vi "Dashboard Main.vi"() -> ()   [LabVIEW 2012]
uses:
  <vilib>/Rock Robotics/WPI/Camera/WPI_CameraWhite Balance Values.ctl
  <vilib>/event_ctls.llb/eventvkey.ctl
  <vilib>/Utility/config.llb/Read Key (String).vi
  <vilib>/Utility/config.llb/Read Key (I32).vi
  <vilib>/Utility/config.llb/Write Key (String).vi
  <vilib>/Utility/config.llb/Write Key (I32).vi
  <vilib>/Utility/config.llb/NI_LVConfig.lvlib
  <vilib>/Utility/inputDevices.llb/joystickAcquire.vi
panel:
  out "Selected Cordinates":i32[](array[numeric])
  out "Latched Cordinates":i32[](array[numeric])
  out "Battery Value":dbl(slide) scale=0.0..14.0 scale format="%#_2e"
  out "Battery":sgl(graph)
  in  "Camera Settings":T1={"Frate Rate"=30, "Compression"=30, "Size"=1} {"Frate Rate" scale=1.0..30.0; "Size" items=["640x480", "320x240", "160x120"]}
  out "Mode":T2(ring)=enum."Auto Disabled"
  out "Camera IP":string
  out "JS1 Z":dbl(slide) scale=-1.0..1.0 scale format="%#_2e"
  out "JS2 Z":dbl(slide) scale=-1.0..1.0 scale format="%#_2e"
  out "Joystick 1":cluster{"X":dbl, "Y":dbl}[](graph)
  out "Joystick 2":cluster{"X":dbl, "Y":dbl}[](graph)
  out "JS Buttons 1":T3
  out "JS Buttons 2":T3
  out "MotorSlide4":dbl(slide) scale=-1.0..1.0 scale format="%#_2e"
  out "MotorSlide3":dbl(slide) scale=-1.0..1.0 scale format="%#_2e"
  out "MotorSlide2":dbl(slide) scale=-1.0..1.0 scale format="%#_2e"
  in  "MotorName3":string="Front Left"
  in  "MotorName4":string="Front Right"
  in  "MotorName1":string="Rear Left"
  in  "MotorName2":string="Rear Right"
  out "MotorChart4":dbl(graph)
  out "MotorChart3":dbl(graph)
  out "MotorChart2":dbl(graph)
  out "MotorSlide1":dbl(slide) scale=-1.0..1.0 scale format="%#_2e"
  out "MotorChart1":dbl(graph)
  out "Robot IP":string
  in  "Dashboard Tab":enum32{"Operation", "Test", "Checklist"}(tab)
  in  "Checkbox 2":bool
  in  "Checkbox 1":bool
  in  "Slider 1":dbl(slide) scale=0.0..100.0
  in  "Slider":dbl(slide) scale=0.0..100.0 scale format="%#_3g"
  in  "On/Off":bool caption="Solenoid"
  in  "Test Name":u16(ring) items=["Select the test to run...", "Example Test", "-------------------------------", "List of tests is built in robot code.", "Replace with your own automated tests."]
  in  "Test Tree":string(tree)
  in  "Motor":cluster{"Value":dbl, "Enable":bool} {"Value" scale=-1.0..1.0 scale format="%#_3g"}
  out "Progress":T4 {"Test Progress" scale=0.0..100.0}
  in  "Rev/Fwd":cluster{"Forward":bool, "Reverse":bool}
  in  "Ring":u16(ring) items=["Auto", "Fixed indoor", "Fixed outdoor 1", "Fixed outdoor 2", "Fixed fluorescent 1", "Fixed fluorescent 2", "Hold current"]
  in  "Listbox":i32(listbox)
  in  "Viewer":enum32{"Camera Image", "Map", "Variables"}(tab)
  out "Mbps":dbl format="%#.1g"
  in  "Enable":bool
  in  "DB Camera Config":bool
  out "Mbps":bool
  out "fps":dbl format="%#.1g"
  out "Image Error Message":string="Timeout in Camera Communications"
  out "Camera Image":T5(plugin-control)
  out "Map":T5(plugin-control)
  out "Distance [Meter]":dbl
  out "Angel [Degrees]":dbl
  in  "Goal Number":i32(knob) scale=1.0..5.0
  out "Tree":string(tree)
  # "Drive & Motors"
  # "Robot IP:"
  # "Customize by placing controls and indicators here and name to match\nDashboard Variables on robot."
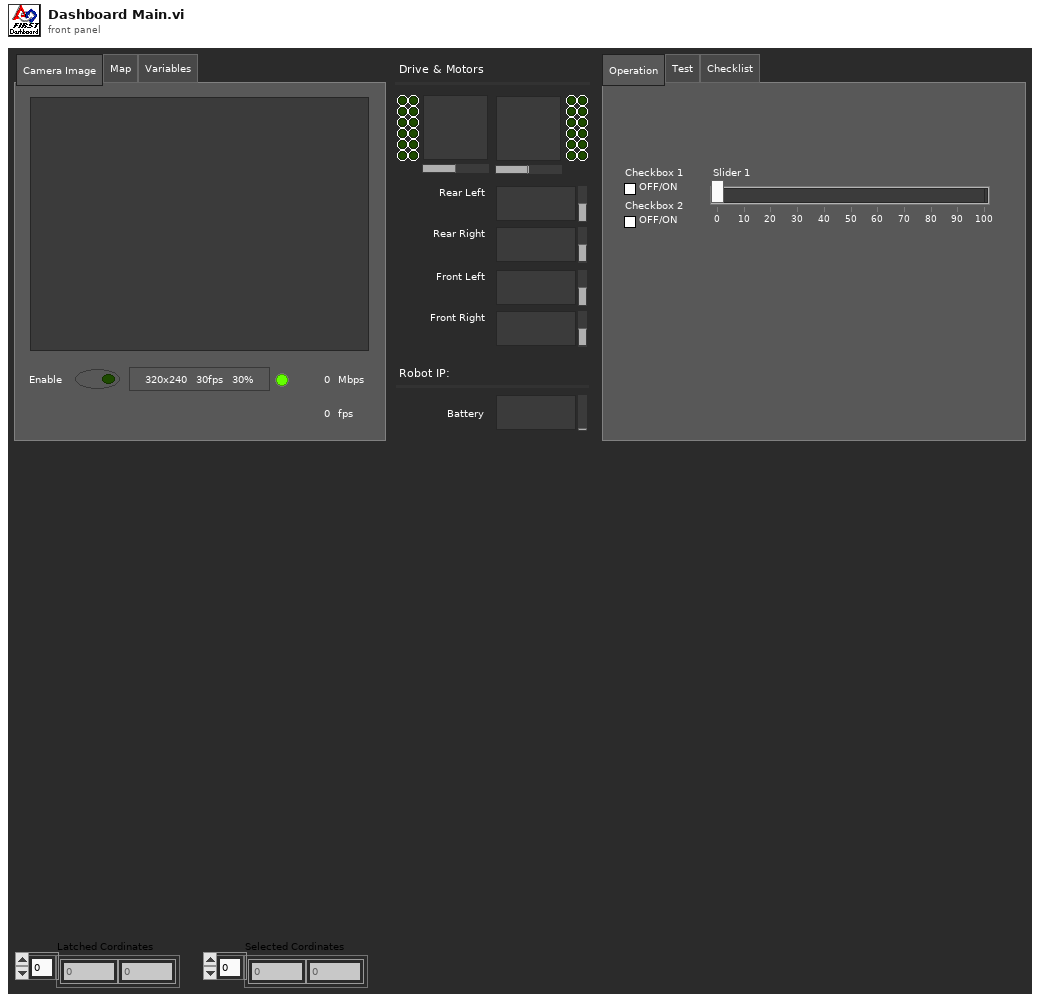
[diagram p1: front panel]
types:
  T1 = cluster{"Frate Rate":i32, "Compression":i32, "Size":u16}
  T2 = enum8{"Tele-Op Disabled", "Tele-Op Enabled", "Auto Disabled", "Auto Enabled", "Test Disabled", "Test Enabled", ""}
  T3 = cluster{bool, bool, bool, bool, bool, bool, bool, bool, bool, bool, bool, bool}
  T4 = cluster{"Test Progress":u8, "Test Progress Text":string}
  T5 = typedef "IMAQ Image.ctl" = refnum<image>
  T6 = typedef "Image Type" = u32
  T7 = typedef "WPI_CameraWhite Balance Values.ctl" = enum16{"Auto", "Fixed indoor", "Fixed outdoor 1", "Fixed outdoor 2", "Fixed fluorescent 1", "Fixed fluorescent 2", "Hold current"}
  T8 = typedef "SkeletonTrackState.ctl" = enum32{"NotTracked", "PositionOnly", "Tracked"}
  T9 = cluster{"TrackingState":u8[], "Position":cluster{"x":sgl, "y":sgl, "z":sgl}, cluster{"x":sgl, "y":sgl, "z":sgl, sgl}[], "TrackState":T8}
  T10 = cluster{cluster{"ScaledToPercentRange":dbl, "ScaledToPercentRange":dbl, "ScaledToPercentRange":dbl}, cluster{bool, bool, bool}}[]
  T11 = cluster{cluster{"ScaledToPercentRange":dbl, "ScaledToPercentRange":dbl, "ScaledToPercentRange":dbl}, cluster{bool, bool, bool}}
  T12 = cluster{"ScaledToPercentRange":dbl, "ScaledToPercentRange":dbl, "ScaledToPercentRange":dbl}
  T13 = typedef "LVRectTypeDef.ctl" = cluster{"Left":i16, "Top":i16, "Right":i16, "Bottom":i16}
  T14 = cluster{"Competition mode":bool, "Robot Link":bool, "Autonomous":bool, "Enabled":bool, "E-Stop":bool, "Simulated":bool, "TestMode":bool, "Docked Window":bool}
  T15 = cluster{"Boolean Array[0]":bool, "Boolean Array[1]":bool, "Boolean Array[2]":bool, "Boolean Array[3]":bool, "Boolean Array[4]":bool, "Boolean Array[5]":bool, "Boolean Array[6]":bool, "Boolean Array[7]":bool, "Boolean Array[8]":bool, "Boolean Array[9]":bool, "Boolean Array[10]":bool, "Boolean Array[11]":bool}
  T16 = cluster{"Coordinates[0]":i32, "Coordinates[1]":i32, "Coordinates[2]":i32, "Coordinates[3]":i32, "Coordinates[4]":i32, "Coordinates[5]":i32, "Coordinates[6]":i32, "Coordinates[7]":i32, "Coordinates[8]":i32}
  T17 = typedef "WPI_CameraDevRef.ctl" = cluster{"Camera Address":string, "CameraStatus":errorcluster, "Acquire Image Notifier":refnum<notifier>}
  T18 = typedef "NI_LVConfig.lvlib/Config Data RefNum.ctl" = refnum<k1>
  T19 = typedef "eventvkey.ctl" = enum16{"ASCII", "Enter", "Return", "Shift", "Ctrl", "Alt", "Cmd", "Opt", "Caps", "NumLock", "Clear", "Break", "Up", "Down", "Left", "Right", "Insert", "Delete", "Home", "End", "PageUp", "PageDown", "Escape", "Help", "Pause", "ScrollLock", "F1", "F2", "F3", "F4", "F5", "F6", "F7", "F8", "F9", "F10", "F11", "F12", "F13", "F14", "F15", "F16", "F17", "F18", "F19", "F20", "F21", "F22", "F23", "F24", "Play", "VolumeUp", "VolumeDown", "Mute", "Two Byte Char"}
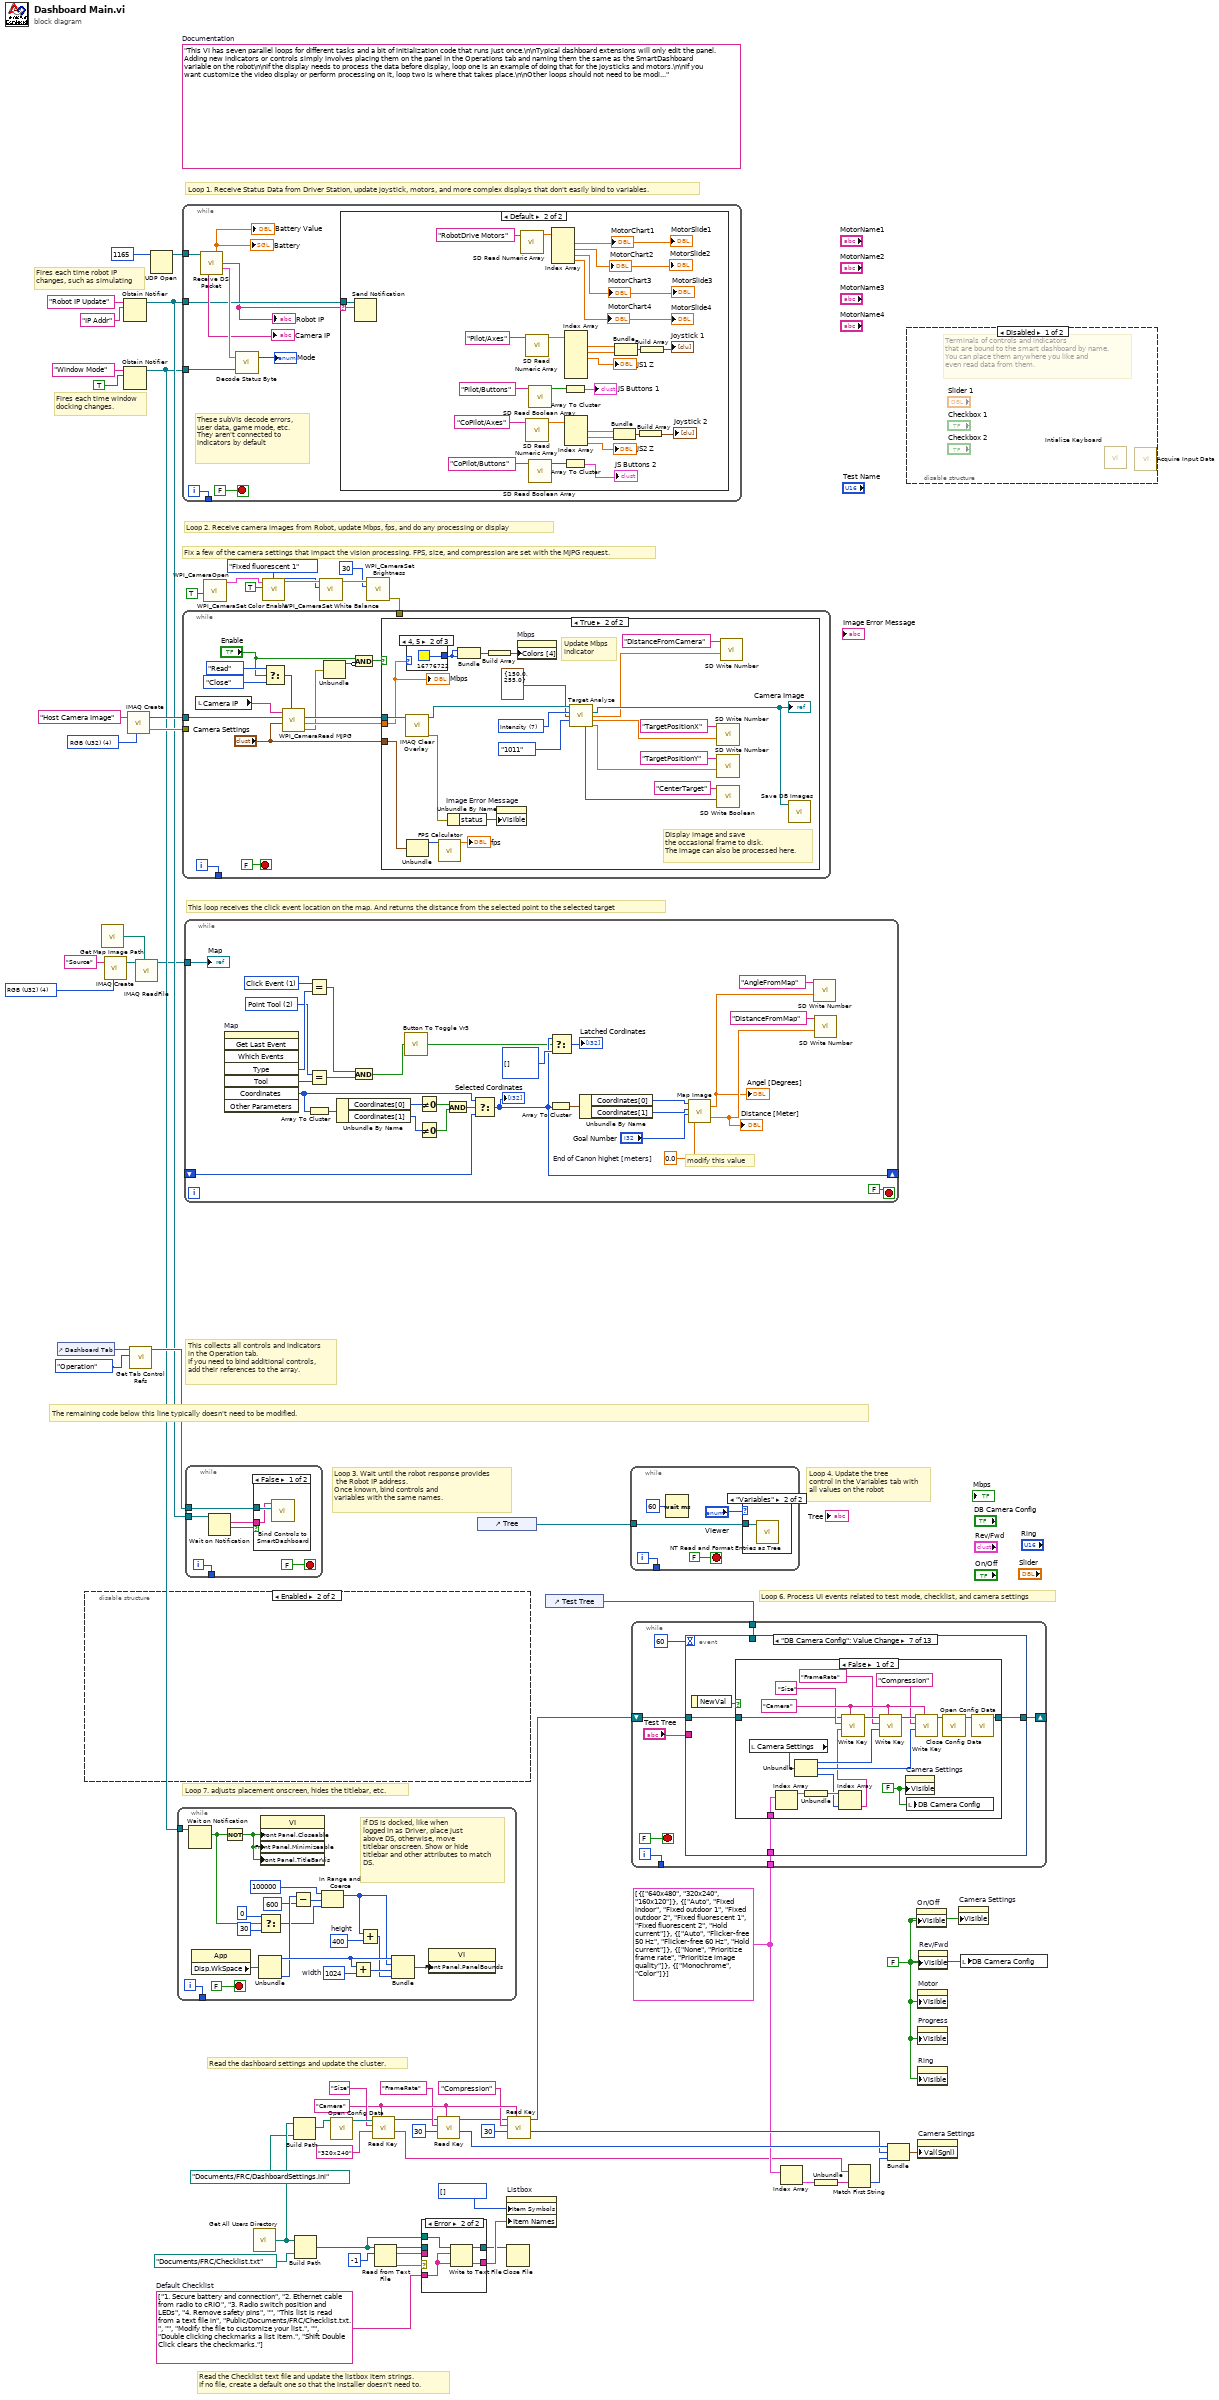
[diagram p0: block diagram]
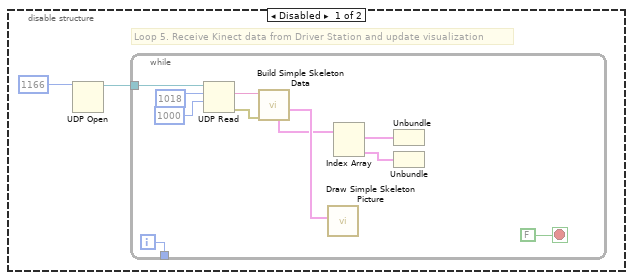
[diagram p2: hidden frame]
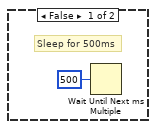
[diagram p5: hidden frame]
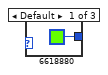
[diagram p6: hidden frame]
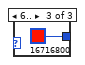
[diagram p7: hidden frame]
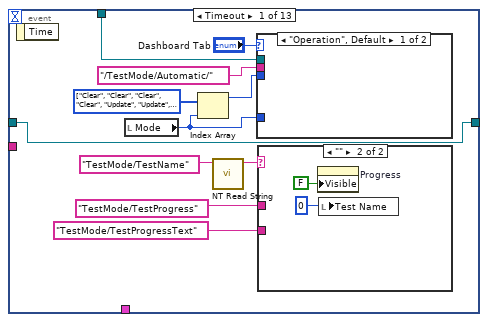
[diagram p9: hidden frame]
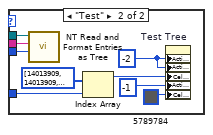
[diagram p10: hidden frame]
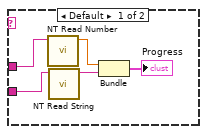
[diagram p11: hidden frame]
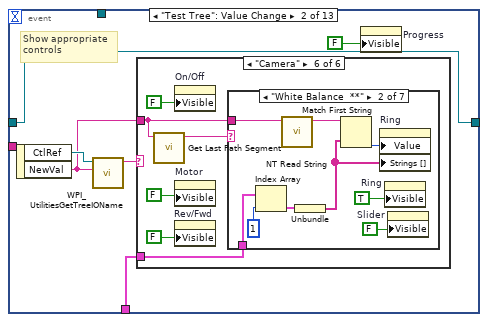
[diagram p12: hidden frame]
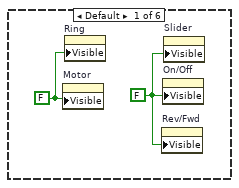
[diagram p13: hidden frame]
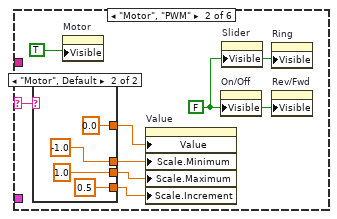
[diagram p14: hidden frame]
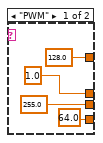
[diagram p15: hidden frame]
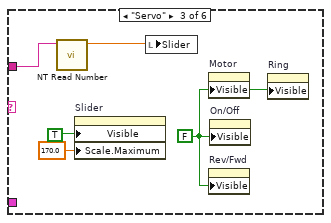
[diagram p16: hidden frame]
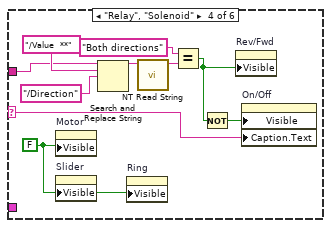
[diagram p17: hidden frame]
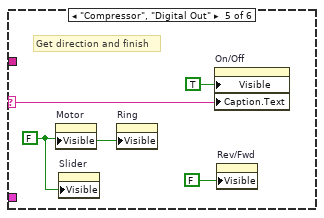
[diagram p18: hidden frame]
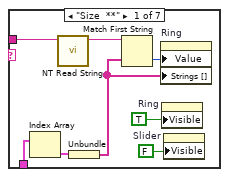
[diagram p19: hidden frame]
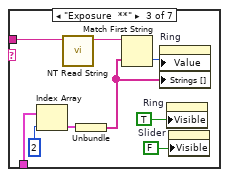
[diagram p20: hidden frame]
diagram:
  w5 = T6 4 items=["Grayscale (U8)", "Grayscale (I16)", "Grayscale (SGL)", "Complex (CSG)", "RGB (U32)", "HSL (U32)", "RGB (U64)", "Grayscale (U16)"] ("Image Type")
  w34 = "Camera"
  w26 = cluster{string[]}[] [{["640x480", "320x240", "160x120"]}, {["Auto", "Fixed indoor", "Fixed outdoor 1", "Fixed outdoor 2", "Fixed fluorescent 1", "Fixed fluorescent 2", "Hold current"]}, {["Auto", "Flicker-free 50 Hz", "Flicker-free 60 Hz", "Hold current"]}, {["None", "Prioritize frame rate", "Prioritize image quality"]}, {["Monochrome", "Color"]}]
  w42 = string[] ["1. Secure battery and connection", "2. Ethernet cable from radio to cRIO", "3. Radio switch position and LEDs", "4. Remove safety pins", "", "This list is read from a text file in", "Public/Documents/FRC/Checklist.txt.", "", "Modify the file to customize your list.", "", "Double clicking checkmarks a list item.", "Shift Double Click clears the checkmarks."]  # Default Checklist
  w40 = FALSE ("Visible")
  (unwired) "This VI has seven parallel loops for different tasks and a bit of initialization code that runs just once.\n\nTypical dashboard extensions will only edit the panel. Adding new indicators or controls simply involves placing them on the panel in the Operations tab and naming them the same as the SmartDashboard variable on the robot\n\nIf the display needs to process the data before display, loop one is an example of doing that for the joysticks and motors.\n\nIf you want customize the video display or perform processing on it, loop two is where that takes place.\n\nOther loops should not need to be modified. They are pretty standard, and document the task they perform."  # Documentation
  w61 = T6 4 items=["Grayscale (U8)", "Grayscale (I16)", "Grayscale (SGL)", "Complex (CSG)", "RGB (U32)", "HSL (U32)", "RGB (U64)"] ("Image Type")
  # "This loop receives the click event location on the map. And returns the distance from the selected point to the selected target"
  # "Fix a few of the camera settings that impact the vision processing. FPS, size, and compression are set with the MJPG request."
  # "Fires each time robot IP\nchanges, such as simulating"
  # "Fires each time window\ndocking changes."
  # "Read the Checklist text file and update the listbox item strings.\nIf no file, create a default one so that the installer doesn't need to."
  # "This collects all controls and indicators\nin the Operation tab.\nIf you need to bind additional controls,\nadd their references to the array."
  # "The remaining code below this line typically doesn't need to be modified."
  # "Loop 6. Process UI events related to test mode, checklist, and camera settings"
  # "Read the dashboard settings and update the cluster."
  # "Loop 4. Update the tree\ncontrol in the Variables tab with\nall values on the robot"
  # "Loop 3. Wait until the robot response provides\n the Robot IP address.\nOnce known, bind controls and\nvariables with the same names."
  # "Loop 7. adjusts placement onscreen, hides the titlebar, etc."
  # "Loop 1. Receive Status Data from Driver Station, update joystick, motors, and more complex displays that don't easily bind to variables."
  # "Loop 2. Receive camera images from Robot, update Mbps, fps, and do any processing or display"
  n1 = control-ref of="Dashboard Tab"() -> (w56:refnum<vi>)
  n2 = disable-structure shown="Enabled" {
    frame Disabled {
      # "Loop 5. Receive Kinect data from Driver Station and update visualization"
      n3 = UDP Open(11:u16 1166 ("port")) -> (port=w64:refnum<k16>)  [unwired: 2 in, 4 out]
      n4 = while {
        tunnel: w64 -> [w80]
        tunnel: [w67] -> _
        i -> [w67]
        stop <- FALSE stop-if-true
        n5 = UDP Read(connection ID=w80, max size (548)=1018 ("bytes to read"), timeout ms (25000)=1000) -> (data out=w75:string, error out=w66:errorcluster)  [unwired: 1 in, 3 out]
        n6 = call "Build Simple Skeleton Data.vi"("error in (no error)"=w66, "data in"=w75) -> ("Skeleton Data"=w76:T9, "NumPlayers"=w78:i8, "Version String"=w79:string, "Simple Joystick Info"=w73:T10)  [unwired: 5 in, 1 out]
        n7 = call "Draw Simple Skeleton Picture.vi"("Simple Skeleton"=w76) -> ("new picture out"=w77:picture)  [unwired: 10 in]
        n8 = Index Array(array=w73) -> (element #1=w72:T11, element #2=w71:T11)  [unwired: 2 in]
        n9 = Unbundle(w72) -> (w70:T12)  [unwired: 1 out]
        n10 = Unbundle(w71) -> (w69:T12, w68:cluster{bool, bool, bool})
      }
    }
    frame Enabled {
    }
  }
  n11 = call "Get Map Image Path.vi"() -> ("Image Path"=w1:path)  [unwired: 1 in]
  n12 = call "IMAQ Create"("Image Name"="Source", "Image Type"=w5) -> ("New Image"=w3:T5)  [unwired: 2 in, 2 out]
  n13 = Obtain Notifier(name (unnamed)="Robot IP Update", notification data type="IP Addr" ("name (unnamed)")) -> (notifier out=w53:refnum<notifier>)  [unwired: 2 in, 2 out]
  n14 = Obtain Notifier(name (unnamed)="Window Mode", notification data type=TRUE) -> (notifier out=w46:refnum<notifier>)  [unwired: 2 in, 2 out]
  n15 = call "IMAQ Create"("Image Name"="Host Camera Image", "Image Type"=w61) -> ("New Image"=w59:T5, "error out"=w58:errorcluster)  [unwired: 2 in, 1 out]
  n16 = call <vilib>:"Get Tab Control Refs.vi"("Page Index"=enum32{"Operation", "Test"}."Operation" ("Dashboard Tab"), "TabControl in"=w56) -> ("ControlsOnPage"=w57:refnum<vi>[])  [unwired: 9 in]
  n17 = call "IMAQ ReadFile"("File Path"=w1, "Image"=w3) -> ("Image Out"=w4:T5)  [unwired: 5 in, 4 out]
  n18 = UDP Open(11:u16 1165 ("port")) -> (port=w62:refnum<k16>)  [unwired: 2 in, 4 out]
  n19 = while {
    tunnel: w46 -> [w101]
    tunnel: [w99] -> _
    i -> [w99]
    stop <- FALSE stop-if-true
    w91 = 1024  # width
    w94 = 400  # height
    # "If DS is docked, like when\nlogged in as Driver, place just\nabove DS, otherwise, move\ntitlebar onscreen. Show or hide\ntitlebar and other attributes to match\nDS."
    n20 = Wait on Notification(notifier=w101) -> (notification=w86:bool)  [unwired: 3 in, 3 out]
    n21 = property class="App"() -> ("Disp.WkSpace"=w97:T13)  [unwired: 2 in, 2 out]
    n22 = Not(x=w86) -> (.not. x?=w100:bool)
    n23 = Unbundle(w97) -> ("Left"=w95:i16, "Bottom"=w92:i16)  [unwired: 2 out]
    n24 = Select(t=0, s=w86, f=30) -> (s? t:f=w85:i32)
    n25 = property class="VI"("Front Panel.Closeable"=w100, "Front Panel.Minimizeable"=w100, "Front Panel.TitleBarVis"=w100) -> ()  [unwired: 2 in, 2 out]
    n26 = Subtract(x=w92, y=600) -> (x-y=w89:i32)
    n27 = In Range and Coerce(upper limit=100000, x=w89, lower limit=w85) -> (coerced(x)=w83:i32)  [unwired: 1 out]
    n28 = Add(x=w95, y=w91) -> (x+y=w96:i32)
    n29 = Add(x=w83, y=w94) -> (x+y=w93:i32)
    n30 = Bundle("Left"=w95, w83, w96, w93) -> (w98:cluster{"Left":i16, i32, i32, i32})  [unwired: 1 out]
    n31 = property class="VI"("Front Panel.PanelBounds"=w98) -> ()  [unwired: 2 in, 2 out]
  }
  n32 = while {
    tunnel: w62 -> [w110]
    tunnel: w53 -> [w104]
    tunnel: w46 -> [w108]
    tunnel: [w105] -> _
    i -> [w105]
    stop <- FALSE stop-if-true
    # "These subVIs decode errors, user data, game mode, etc.\nThey aren't connected to indicators by default"
    n33 = call "Receive DS Packet.vi"("Recv Socket"=w110) -> ("Battery"=→"Battery" →"Battery Value":sgl, "Robot IP Address"=w103:string, "Status"=w111:T14, "Camera IP Address"=→"Camera IP":string)  [unwired: 1 in, 10 out]
    "Robot IP" <- w103
    n34 = call "Decode Status Byte.vi"("Window Mode Notifier"=w108, "Status"=w111) -> ("Mode"=→"Mode":T2)  [unwired: 1 out]
    n35 = case shown="Default" w103 {
      selector: w103 -> [_ w113]
      tunnel: w104 -> [_ w114]
      frame "0.0.0.0" {
        # "Robot not responding, don't poll the variables"
      }
      frame Default {
        n36 = Send Notification(notification=w113, notifier=w114) -> ()  [unwired: 1 in, 2 out]
        n37 = call <vilib>:"SD Read Numeric Array.vi"("Name"="RobotDrive Motors") -> ("Numeric Array"=w137:dbl[])  [unwired: 8 in, 2 out]
        n38 = call <vilib>:"SD Read Numeric Array.vi"("Name"="Pilot/Axes") -> ("Numeric Array"=w130:dbl[])  [unwired: 8 in, 2 out]
        n39 = call <vilib>:"SD Read Numeric Array.vi"("Name"="CoPilot/Axes") -> ("Numeric Array"=w124:dbl[])  [unwired: 8 in, 2 out]
        n40 = call <vilib>:"SD Read Boolean Array.vi"("Name"="Pilot/Buttons") -> ("Boolean Array"=w132:bool[])  [unwired: 8 in, 2 out]
        n41 = call <vilib>:"SD Read Boolean Array.vi"("Name"="CoPilot/Buttons") -> ("Boolean Array"=w123:bool[])  [unwired: 8 in, 2 out]
        n42 = Index Array(array=w137) -> (element #1=→"MotorChart1" →"MotorSlide1":dbl, element #2=→"MotorSlide2" →"MotorChart2":dbl, element #3=→"MotorChart3" →"MotorSlide3":dbl, element #4=→"MotorChart4" →"MotorSlide4":dbl)  [unwired: 4 in]
        n43 = Array To Cluster(array=w132) -> (cluster=→"JS Buttons 1":T15)
        n44 = Array To Cluster(array=w123) -> (cluster=→"JS Buttons 2":T15)
        n45 = Index Array(array=w130) -> (element #1=w127:dbl, element #2=w128:dbl, element #3=→"JS1 Z":dbl)  [unwired: 6 in, 3 out]
        n46 = Index Array(array=w124) -> (element #1=w119:dbl, element #2=w118:dbl, element #3=→"JS2 Z":dbl)  [unwired: 3 in]
        n47 = Bundle("Numeric"=w119, "Numeric"=w118) -> (w120:cluster{"Numeric":dbl, "Numeric":dbl})  [unwired: 1 in]
        n48 = Bundle("Numeric"=w127, "Numeric"=w128) -> (w126:cluster{"Numeric":dbl, "Numeric":dbl})  [unwired: 1 in]
        n49 = Build Array(w120) -> (→"Joystick 2":cluster{"Numeric":dbl, "Numeric":dbl}[])
        n50 = Build Array(w126) -> (→"Joystick 1":cluster{"Numeric":dbl, "Numeric":dbl}[])
      }
    }
  }
  n51 = while {
    tunnel: w4 -> [w164]
    shift-right: [w151] -> _
    shift-left: _ -> [w155]
    stop <- FALSE stop-if-true
    w145 = 0.0  # End of Canon highet [meters]
    w165 = 2 items=["None", "Selection Tool", "Point Tool", "Line Tool", "Rectangle Tool", "Oval Tool", "Polygon Tool", "ClosedFreehandTool", "Annulus Tool", "Rotated Rectangle Tool", "Zoom Tool", "Pan Tool", "Polyline Tool", "Freehand Tool"] ("Tool")
    w166 = 1 items=["No Event"=0, "Click Event"=1, "Draw Event"=2, "Size Event"=4, "Scroll Event"=5, "Double Click Event"=8] ("Type")
    # "modify this value"
    n52 = invoke on="Map" class="ImageControl" method="Get Last Event"() -> ("Type"=w167:i32, "Tool"=w170:i32, "Coordinates"=w156:i32[])  [unwired: 8 in, 5 out]
    n53 = Equal?(x=w166, y=w167) -> (x = y?=w168:bool)
    n54 = Equal?(x=w165, y=w170) -> (x = y?=w169:bool)
    n55 = Array To Cluster(array=w156) -> (cluster=w162:T16)
    n56 = Unbundle By Name(w162) -> ("Coordinates[0]"=w160:i32, "Coordinates[1]"=w158:i32)
    n57 = And(x=w168, y=w169) -> (x .and. y?=w150:bool)
    n58 = call "Button To Toggle Vr3.vi"("InValue"=w150) -> ("Result"=w149:bool)
    n59 = Not Equal To 0?(x=w160) -> (x != 0?=w161:bool)
    n60 = Not Equal To 0?(x=w158) -> (x != 0?=w159:bool)
    n61 = And(x=w161, y=w159) -> (x .and. y?=w157:bool)
    n62 = Select(t=w156, s=w157, f=w155) -> (s? t:f=w151:i32[])
    "Selected Cordinates" <- w151
    n63 = Array To Cluster(array=w151) -> (cluster=w152:T16)
    n64 = Select(t=w151, s=w149, f=i32[] [] ("Coordinates")) -> (s? t:f=→"Latched Cordinates":i32[])
    n65 = Unbundle By Name(w152) -> ("Coordinates[0]"=w147:i32, "Coordinates[1]"=w148:i32)
    n66 = call "Map Image.vi"("End of Canon highet [meters]"=w145, "Goal Number"="Goal Number", "Y[Pixels]"=w148, "X [Pixels]"=w147) -> ("Distance [Meter]"=w142:dbl, "Angel [Degrees]"=w141:dbl)
    "Distance [Meter]" <- w142
    "Angel [Degrees]" <- w141
    n67 = call <vilib>:"SD Write Number.vi"("Numeric"=w141, "Name"="AngleFromMap") -> ()  [unwired: 8 in, 2 out]
    n68 = call <vilib>:"SD Write Number.vi"("Numeric"=w142, "Name"="DistanceFromMap") -> ()  [unwired: 8 in, 2 out]
    "Map" <- w164
  }
  n69 = while {
    tunnel: w57 -> [w176]
    tunnel: w53 -> [w173]
    tunnel: [w171] -> _
    i -> [w171]
    stop <- FALSE stop-if-true
    n70 = Wait on Notification(notifier=w173) -> (notification=w172:string, timed out?=w174:bool)  [unwired: 3 in, 2 out]
    n71 = case shown="False" w174 {
      tunnel: w176 -> [w178 _]
      tunnel: w172 -> [w177 _]
      frame False {
        n72 = call <vilib>:"Bind Controls to SmartDashboard.vi"("Bound Control Refs"=w178, "Server IP Address"=w177) -> ()  [unwired: 10 in]
      }
      frame True {
      }
    }
  }
  n73 = call <vilib>:"WPI_CameraOpen.vi"("Disallow Simulation"=TRUE) -> ("CameraDevRef"=w13:T17)  [unwired: 9 in, 1 out]
  n74 = call "Get All Users Directory.vi"() -> ("All User Path"=w39:path)
  n75 = call <vilib>:"WPI_CameraSet Color Enable.vi"("Color Enabled"=TRUE, "CameraDevRef"=w13) -> ("CameraDevRef Out"=w11:T17)  [unwired: 8 in, 1 out]
  n76 = Build Path(base path=w39, name or relative path=path "Documents/FRC/DashboardSettings.ini") -> (appended path=w38:path)
  n77 = Build Path(base path=w39, name or relative path=path "Documents/FRC/Checklist.txt") -> (appended path=w43:path)
  n78 = call <vilib>:"WPI_CameraSet White Balance.vi"("White Balance"=WPI_CameraWhite_Balance_Values."Fixed fluorescent 1", "CameraDevRef"=w11) -> ("CameraDevRef Out"=w9:T17)  [unwired: 8 in, 1 out]
  n79 = call <vilib>:"Open Config Data.vi"("configuration file path"=w38) -> ("refnum"=w37:T18)  [unwired: 8 in, 2 out]
  n80 = call <vilib>:"WPI_CameraSet Brightness.vi"("Brightness"=30, "CameraDevRef"=w9) -> ("error out"=w6:errorcluster)  [unwired: 8 in, 1 out]
  n81 = while {
    tunnel: w59 -> [w188]
    tunnel: w58 -> [_]
    tunnel: [w191] -> _
    tunnel: w6 -> [_]
    i -> [w191]
    stop <- FALSE stop-if-true
    n82 = local read "Camera IP"() -> (w190:string)
    n83 = Select(t=enum16{"Read", "Reopen", "Close"}."Read" ("Operation"), s="Enable", f=enum16{"Read", "Reopen", "Close"}."Close" ("Operation")) -> (s? t:f=w183:enum16{"Read", "Reopen", "Close"})
    n84 = call <vilib>:"WPI_CameraRead MJPG.vi"("Operation"=w183, "Camera Settings"="Camera Settings", "Image"=w188, "address"=w190) -> ("error out"=w182:errorcluster, "Bandwidth (kbps)"=w186:dbl, "Image Out"=w187:T5)  [unwired: 5 in]
    n85 = Unbundle(w182) -> ("status"=w180:bool)  [unwired: 2 out]
    n86 = Compound Arithmetic op=AND("Enable", invert w180) -> (w179:bool)
    n87 = case shown="True" w179 {
      tunnel: "Camera Settings" -> [_ w208]
      tunnel: w187 -> [_ w211]
      tunnel: w186 -> [_ w210]
      frame False {
        # "Sleep for 500ms"
        n88 = Wait Until Next ms Multiple(millisecond multiple=u32 500) -> ()  [unwired: 1 out]
      }
      frame True {
        w200 = 7 items=["Red", "Green", "Blue", "Hue", "Saturation", "Luminance", "Value", "Intensity"] ("Color Plane")
        # "Display image and save\nthe occasional frame to disk.\nThe image can also be processed here."
        # "Update Mbps\nindicator"
        n89 = call "IMAQ Clear Overlay"("Image"=w211) -> ("error out"=w215:errorcluster, "Image Out"=w206:T5)  [unwired: 2 in, 7 out]
        n90 = case shown="4, 5" w210 {
          tunnel: [u32 6618880 ("Color Box") u32 16776722 ("Color Box") u32 16716800 ("Color Box")] -> w212
          frame Default {
          }
          frame 4, 5 {
          }
          frame 6.. {
          }
        }
        n91 = Unbundle(w208) -> ("Frate Rate"=w207:i32)  [unwired: 2 out]
        n92 = call "FPS Calculator.vi"("Average Count"=w207) -> ("fps"=→"fps":dbl)  [unwired: 10 in]
        n93 = Unbundle By Name(w215) -> ("status"=w216:bool)
        n94 = Bundle("Color Box"=w212, "Color Box"=w212) -> (w214:cluster{"Color Box":u32, "Color Box":u32})  [unwired: 1 out]
        n95 = Build Array(w214) -> (w213:cluster{"Color Box":u32, "Color Box":u32}[])
        n96 = property on="Image Error Message" class="Str"("Visible"=w216) -> ()  [unwired: 2 in, 2 out]
        n97 = property on="Mbps" class="Bool (strict)"("Colors [4]"=w213) -> ()  [unwired: 2 in, 2 out]
        n98 = call "Target Analyze.vi"("Original Image_in"=w206, "Color Plane"=w200, "Range"=cluster{"Lower value":sgl, "Upper value":sgl} {"Lower value"=150.0, "Upper value"=255.0}, "Camera Type"=enum16{"206", "1011"}."1011") -> ("Processed Image"=w205:T5, "Distance [m]"=w196:dbl, "Position of Target Center X"=w195:dbl, "Center Target"=w197:bool, "Position of Target Center Y"=w194:dbl)  [unwired: 5 in, 2 out]
        "Camera Image" <- w205
        n99 = call <vilib>:"SD Write Number.vi"("Numeric"=w195, "Name"="TargetPositionX") -> ()  [unwired: 8 in, 2 out]
        n100 = call <vilib>:"SD Write Number.vi"("Numeric"=w194, "Name"="TargetPositionY") -> ()  [unwired: 8 in, 2 out]
        n101 = call <vilib>:"SD Write Boolean.vi"("Boolean"=w197, "Name"="CenterTarget") -> ()  [unwired: 8 in, 2 out]
        n102 = call <vilib>:"SD Write Number.vi"("Numeric"=w196, "Name"="DistanceFromCamera") -> ()  [unwired: 8 in, 2 out]
        n103 = call "Save DB Images.vi"("Image"=w205) -> ()  [unwired: 2 in, 1 out]
        "Mbps" <- w210
      }
    }
  }
  n104 = call-poly <vilib>:"Read Key.vi"("section"=w34, "default value"="320x240", "key"="Size", "refnum"=w37) -> ("value"=w24:string, "refnum out"=w19:T18)  [unwired: 2 in, 4 out]
  n105 = Read from Text File(file (use dialog)=w43, count=-1 ("timeout ms (25000)")) -> (refnum out=w21:refnum<file>, text=w44:string[], error out=w45:errorcluster)  [unwired: 2 in, 1 out]
  n106 = case shown="Error" w45 {
    tunnel: w44 -> [w221 _]
    tunnel: [w221 w223] -> w41
    tunnel: w42 -> [_ w223]
    tunnel: w43 -> [_ w224]
    tunnel: [w220 w222] -> w20
    tunnel: w21 -> [w220 _]
    frame No Error {
    }
    frame Error {
      n107 = Write to Text File(file (use dialog)=w224, text=w223) -> (refnum out=w222:refnum<file>)  [unwired: 2 in, 2 out]
    }
  }
  n108 = call-poly <vilib>:"Read Key.vi"("section"=w34, "default value"=30, "key"="FrameRate", "refnum"=w19) -> ("value"=w29:i32, "refnum out"=w18:T18)  [unwired: 1 in, 5 out]
  n109 = control-ref of="Tree"() -> (w15:refnum<vi>)
  n110 = property on="Listbox" class="LstBox (strict)"("Item Symbols"=i32[] [], "Item Names"=w41) -> ()  [unwired: 2 in, 2 out]
  n111 = Close File(refnum=w20) -> ()  [unwired: 1 in, 2 out]
  n112 = call-poly <vilib>:"Read Key.vi"("section"=w34, "default value"=30, "key"="Compression", "refnum"=w18) -> ("value"=w28:i32, "refnum out"=w16:T18)  [unwired: 1 in, 5 out]
  n113 = control-ref of="Test Tree"() -> (w14:refnum<vi>)
  n114 = while {
    tunnel: [w226] -> _
    tunnel: w15 -> [w225]
    i -> [w226]
    stop <- FALSE stop-if-true
    n115 = Wait (ms)(milliseconds to wait=u32 60) -> ()  [unwired: 1 out]
    n116 = case shown="\"Variables\"" "Viewer" {
      tunnel: w225 -> [_ w230]
      frame Default {
      }
      frame "Variables" {
        n117 = call <vilib>:"NT Read and Format Entries as Tree.vi"("Tree Refnum"=w230) -> ()  [unwired: 9 in, 2 out]
      }
    }
  }
  n118 = while {
    tunnel: w26 -> [w235]
    shift-right: [w234] -> _
    shift-left: w16 -> [w233]
    tunnel: [w232] -> _
    tunnel: w14 -> [w231]
    i -> [w232]
    stop <- FALSE stop-if-true
    n119 = event shown="[6] \"DB Camera Config\": Value Change" {
      selector: _ -> [_ _ _ _ _ _ _ _ _ _ _ _ _]
      dyn-events: _ -> [_ _ _ _ _ _ _ _ _ _ _ _ _]
      timeout: u32 60 ("milliseconds to wait") -> [_ _ _ _ _ _ _ _ _ _ _ _ _]
      tunnel: w231 -> [w245 _ _ _ _ _ _ _ _ _ _ _ _]
      tunnel: "Test Tree" -> [_ _ _ _ _ _ _ _ w439 w447 w449 w453 w461]
      tunnel: w235 -> [_ w267 _ _ _ _ w403 w433 _ _ _ _ _]
      tunnel: [w239 w266 _ w369 w377 w389 w402 w426 w438 w445 w448 w452 w460] -> w234
      tunnel: w233 -> [w239 w266 _ w369 w377 w389 w401 w426 w438 w445 w448 w452 w460]
      event Timeout {
        w244 = enum16{"Update", "Clear"}[] [enum."Clear", enum."Clear", enum."Clear", enum."Clear", enum."Update", enum."Update", enum."Clear"] items=["Update", "Clear"]
        n120 = event-data() -> ()  [unwired: 1 in, 1 out]
        n121 = local read "Mode"() -> (w242:T2)
        n122 = Index Array(array=w244, index=w242) -> (element=w243:enum16{"Update", "Clear"})
        n123 = call <vilib>:"NT Read String.vi"("Name"="TestMode/TestName") -> ("String"=w248:string)  [unwired: 9 in, 1 out]
        n124 = case shown="\"Operation\", Default" "Dashboard Tab" {
          tunnel: w245 -> [_ w258]
          tunnel: "/TestMode/Automatic/" ("Name Pattern") -> [_ w257]
          tunnel: w243 -> [_ w256]
          tunnel: w242 -> [_ w254]
          frame "Operation", Default {
          }
          frame "Test" {
            w253 = -2 ("Active Item:Row Number")
            n125 = call <vilib>:"NT Read and Format Entries as Tree.vi"("Operation"=w256, "Name Pattern"=w257, "Tree Refnum"=w258) -> ()  [unwired: 7 in, 2 out]
            n126 = Index Array(array=u32[] [14013909, 14013909, 14013909, 14013909, 14013909, 16777215, 14013909], index=w254) -> (element=w252:u32)
            n127 = property on="Test Tree" class="Tree (strict)"("Active Item Row Number"=w253, "ActiveColNum"=w253, "CellBG"=w252, "Active Item Row Number"=-1 ("Active Item:Row Number"), "CellBG"=u32 5789784 ("Color Box")) -> ()  [unwired: 2 in, 2 out]
          }
        }
        n128 = case shown="\"\"" w248 {
          tunnel: "TestMode/TestProgress" ("Name") -> [w260 _]
          tunnel: "TestMode/TestProgressText" ("Name") -> [w259 _]
          frame Default {
            n129 = call <vilib>:"NT Read Number.vi"("Name"=w260) -> ("Numeric"=w261:dbl)  [unwired: 9 in, 1 out]
            n130 = call <vilib>:"NT Read String.vi"("Name"=w259) -> ("String"=w262:string)  [unwired: 9 in, 1 out]
            n131 = Bundle("Numeric"=w261, "String"=w262) -> (→"Progress":cluster{"Numeric":dbl, "String":string})  [unwired: 1 in]
          }
          frame "" {
            n132 = property on="Progress" class="Clust (strict)"("Visible"=FALSE) -> ()  [unwired: 2 in, 2 out]
            n133 = local write "Test Name"(u16 0) -> ()
          }
        }
      }
      event "Test Tree": Value Change {
        # "Show appropriate\ncontrols"
        n134 = event-data() -> ("CtlRef"=w270:refnum<vi>, "NewVal"=w268:string)  [unwired: 1 in]
        n135 = call <vilib>:"WPI_UtilitiesGetTreeIOName.vi"("NewVal"=w268, "TreeControl in"=w270) -> ("I/O Name"=w271:string)  [unwired: 9 in]
        n136 = case shown="\"Camera\"" w271 {
          selector: w271 -> [_ w278 _ w296 w305 _]
          tunnel: w268 -> [_ _ w293 w295 _ w312]
          tunnel: w267 -> [_ _ _ _ _ w311]
          frame Default {
            w273 = FALSE ("Visible")
            w272 = FALSE ("Visible")
            n137 = property on="Motor" class="Clust (strict)"("Visible"=w272) -> ()  [unwired: 2 in, 2 out]
            n138 = property on="Ring" class="Ring (strict)"("Visible"=w272) -> ()  [unwired: 2 in, 2 out]
            n139 = property on="Rev/Fwd" class="Clust (strict)"("Visible"=w273) -> ()  [unwired: 2 in, 2 out]
            n140 = property on="On/Off" class="Bool (strict)"("Visible"=w273) -> ()  [unwired: 2 in, 2 out]
            n141 = property on="Slider" class="Slide (strict)"("Visible"=w273) -> ()  [unwired: 2 in, 2 out]
          }
          frame "Motor", "PWM" {
            w279 = FALSE ("Visible")
            n142 = case shown="\"Motor\", Default" w278 {
              tunnel: [1.0 ("Value") -1.0 ("Value")] -> w277
              tunnel: [255.0 ("Value") 1.0 ("Value")] -> w276
              tunnel: [128.0 ("Value") 0.0 ("Value")] -> w275
              tunnel: [64.0 ("Value") 0.5 ("Value")] -> w274
              frame "PWM" {
              }
              frame "Motor", Default {
              }
            }
            n143 = property on="Motor" class="Clust (strict)"("Visible"=TRUE) -> ()  [unwired: 2 in, 2 out]
            n144 = property on="Value" class="Slide (strict)"("Value"=w275, "Scale.Minimum"=w277, "Scale.Maximum"=w276, "Scale.Increment"=w274) -> ()  [unwired: 2 in, 2 out]
            n145 = property on="On/Off" class="Bool (strict)"("Visible"=w279) -> ()  [unwired: 2 in, 2 out]
            n146 = property on="Slider" class="Slide (strict)"("Visible"=w279) -> ()  [unwired: 2 in, 2 out]
            n147 = property on="Ring" class="Ring (strict)"("Visible"=w279) -> ()  [unwired: 2 in, 2 out]
            n148 = property on="Rev/Fwd" class="Clust (strict)"("Visible"=w279) -> ()  [unwired: 2 in, 2 out]
          }
          frame "Servo" {
            w291 = FALSE ("Visible")
            n149 = call <vilib>:"NT Read Number.vi"("Name"=w293) -> ("Numeric"=w292:dbl)  [unwired: 9 in, 1 out]
            n150 = property on="Slider" class="Slide (strict)"("Visible"=TRUE, "Scale.Maximum"=170.0 ("Scale.Range:Maximum")) -> ()  [unwired: 2 in, 2 out]
            n151 = local write "Slider"(w292) -> ()
            n152 = property on="Motor" class="Clust (strict)"("Visible"=w291) -> ()  [unwired: 2 in, 2 out]
            n153 = property on="Rev/Fwd" class="Clust (strict)"("Visible"=w291) -> ()  [unwired: 2 in, 2 out]
            n154 = property on="On/Off" class="Bool (strict)"("Visible"=w291) -> ()  [unwired: 2 in, 2 out]
            n155 = property on="Ring" class="Ring (strict)"("Visible"=w291) -> ()  [unwired: 2 in, 2 out]
          }
          frame "Relay", "Solenoid" {
            w294 = FALSE ("Visible")
            n156 = property on="Motor" class="Clust (strict)"("Visible"=w294) -> ()  [unwired: 2 in, 2 out]
            n157 = property on="Slider" class="Slide (strict)"("Visible"=w294) -> ()  [unwired: 2 in, 2 out]
            n158 = Search and Replace String(input string=w295, search string="/Value  **", replace string="/Direction") -> (result string=w301:string)  [unwired: 5 in, 3 out]
            n159 = property on="Ring" class="Ring (strict)"("Visible"=w294) -> ()  [unwired: 2 in, 2 out]
            n160 = call <vilib>:"NT Read String.vi"("Name"=w301) -> ("String"=w299:string)  [unwired: 9 in, 1 out]
            n161 = Equal?(x="Both directions", y=w299) -> (x = y?=w297:bool)
            n162 = Not(x=w297) -> (.not. x?=w298:bool)
            n163 = property on="Rev/Fwd" class="Clust (strict)"("Visible"=w297) -> ()  [unwired: 2 in, 2 out]
            n164 = property on="On/Off" class="Bool (strict)"("Visible"=w298, "Caption.Text"=w296) -> ()  [unwired: 2 in, 2 out]
          }
          frame "Compressor", "Digital Out" {
            w304 = FALSE ("Visible")
            # "Get direction and finish"
            n165 = property on="Motor" class="Clust (strict)"("Visible"=w304) -> ()  [unwired: 2 in, 2 out]
            n166 = property on="Slider" class="Slide (strict)"("Visible"=w304) -> ()  [unwired: 2 in, 2 out]
            n167 = property on="Ring" class="Ring (strict)"("Visible"=w304) -> ()  [unwired: 2 in, 2 out]
            n168 = property on="On/Off" class="Bool (strict)"("Visible"=TRUE, "Caption.Text"=w305) -> ()  [unwired: 2 in, 2 out]
            n169 = property on="Rev/Fwd" class="Clust (strict)"("Visible"=FALSE) -> ()  [unwired: 2 in, 2 out]
          }
          frame "Camera" {
            n170 = call <vilib>:"Get Last Path Segment.vi"("String in"=w312) -> ("String out"=w313:string)  [unwired: 10 in]
            n171 = property on="On/Off" class="Bool (strict)"("Visible"=FALSE) -> ()  [unwired: 2 in, 2 out]
            n172 = property on="Motor" class="Clust (strict)"("Visible"=FALSE) -> ()  [unwired: 2 in, 2 out]
            n173 = property on="Rev/Fwd" class="Clust (strict)"("Visible"=FALSE) -> ()  [unwired: 2 in, 2 out]
            n174 = case shown="\"White Balance  **\"" w313 {
              tunnel: w312 -> [w319 w328 w337 w346 w355 _ w361]
              tunnel: w311 -> [w317 w325 w334 w343 w352 _ _]
              frame "Size  **" {
                n175 = Index Array(array=w317) -> (element=w316:cluster{string[]})  [unwired: 1 in]
                n176 = call <vilib>:"NT Read String.vi"("Name"=w319) -> ("String"=w318:string)  [unwired: 9 in, 1 out]
                n177 = Unbundle(w316) -> (w314:string[])
                n178 = Match First String(2:w314, 3:w318) -> (0:w315:i32)  [unwired: 1 out]
                n179 = property on="Ring" class="Ring (strict)"("Value"=w315, "Strings []"=w314) -> ()  [unwired: 2 in, 2 out]
                n180 = property on="Ring" class="Ring (strict)"("Visible"=TRUE) -> ()  [unwired: 2 in, 2 out]
                n181 = property on="Slider" class="Slide (strict)"("Visible"=FALSE) -> ()  [unwired: 2 in, 2 out]
              }
              frame "White Balance  **" {
                n182 = Index Array(array=w325, index=1) -> (element=w326:cluster{string[]})
                n183 = call <vilib>:"NT Read String.vi"("Name"=w328) -> ("String"=w327:string)  [unwired: 9 in, 1 out]
                n184 = Unbundle(w326) -> (w323:string[])
                n185 = Match First String(2:w323, 3:w327) -> (0:w322:i32)  [unwired: 1 out]
                n186 = property on="Ring" class="Ring (strict)"("Value"=w322, "Strings []"=w323) -> ()  [unwired: 2 in, 2 out]
                n187 = property on="Ring" class="Ring (strict)"("Visible"=TRUE) -> ()  [unwired: 2 in, 2 out]
                n188 = property on="Slider" class="Slide (strict)"("Visible"=FALSE) -> ()  [unwired: 2 in, 2 out]
              }
              frame "Exposure  **" {
                n189 = Index Array(array=w334, index=2) -> (element=w335:cluster{string[]})
                n190 = call <vilib>:"NT Read String.vi"("Name"=w337) -> ("String"=w336:string)  [unwired: 9 in, 1 out]
                n191 = Unbundle(w335) -> (w331:string[])
                n192 = Match First String(2:w331, 3:w336) -> (0:w332:i32)  [unwired: 1 out]
                n193 = property on="Ring" class="Ring (strict)"("Value"=w332, "Strings []"=w331) -> ()  [unwired: 2 in, 2 out]
                n194 = property on="Ring" class="Ring (strict)"("Visible"=TRUE) -> ()  [unwired: 2 in, 2 out]
                n195 = property on="Slider" class="Slide (strict)"("Visible"=FALSE) -> ()  [unwired: 2 in, 2 out]
              }
              frame "Exposure Priority  **" {
                n196 = Index Array(array=w343, index=3) -> (element=w344:cluster{string[]})
                n197 = call <vilib>:"NT Read String.vi"("Name"=w346) -> ("String"=w345:string)  [unwired: 9 in, 1 out]
                n198 = Unbundle(w344) -> (w340:string[])
                n199 = Match First String(2:w340, 3:w345) -> (0:w341:i32)  [unwired: 1 out]
                n200 = property on="Ring" class="Ring (strict)"("Value"=w341, "Strings []"=w340) -> ()  [unwired: 2 in, 2 out]
                n201 = property on="Ring" class="Ring (strict)"("Visible"=TRUE) -> ()  [unwired: 2 in, 2 out]
                n202 = property on="Slider" class="Slide (strict)"("Visible"=FALSE) -> ()  [unwired: 2 in, 2 out]
              }
              frame "Color Enable  **" {
                n203 = Index Array(array=w352, index=4) -> (element=w353:cluster{string[]})
                n204 = call <vilib>:"NT Read String.vi"("Name"=w355) -> ("String"=w354:string)  [unwired: 9 in, 1 out]
                n205 = Unbundle(w353) -> (w349:string[])
                n206 = Match First String(2:w349, 3:w354) -> (0:w350:i32)  [unwired: 1 out]
                n207 = property on="Ring" class="Ring (strict)"("Value"=w350, "Strings []"=w349) -> ()  [unwired: 2 in, 2 out]
                n208 = property on="Ring" class="Ring (strict)"("Visible"=TRUE) -> ()  [unwired: 2 in, 2 out]
                n209 = property on="Slider" class="Slide (strict)"("Visible"=FALSE) -> ()  [unwired: 2 in, 2 out]
              }
              frame Default {
                n210 = property on="Ring" class="Ring (strict)"("Visible"=FALSE) -> ()  [unwired: 2 in, 2 out]
                n211 = property on="Slider" class="Slide (strict)"("Visible"=FALSE) -> ()  [unwired: 2 in, 2 out]
              }
              frame "Brightness  **", "Color Level  **", "Compression  **", "FPS  **", "Sharpness  **" {
                n212 = call <vilib>:"NT Read Number.vi"("Name"=w361) -> ("Numeric"=w360:dbl)  [unwired: 9 in, 1 out]
                n213 = local write "Slider"(w360) -> ()
                n214 = property on="Slider" class="Slide (strict)"("Visible"=TRUE, "Scale.Maximum"=100.0 ("Scale.Range:Maximum")) -> ()  [unwired: 2 in, 2 out]
                n215 = property on="Ring" class="Ring (strict)"("Visible"=FALSE) -> ()  [unwired: 2 in, 2 out]
              }
            }
          }
        }
        n216 = property on="Progress" class="Clust (strict)"("Visible"=FALSE) -> ()  [unwired: 2 in, 2 out]
      }
      event "Test Name": Mouse Enter {
        # "Populate the ring with the list of tests"
        n217 = event-data() -> ()  [unwired: 1 in, 1 out]
        n218 = call <vilib>:"NT Read String Array.vi"("Name"="TestMode/TestList") -> ("String Array"=w368:string[])  [unwired: 9 in, 1 out]
        n219 = Build Array (concatenate)("Select the test to run...", w368) -> (w367:string[])
        n220 = property on="Test Name" class="Ring (strict)"("Strings []"=w367) -> ()  [unwired: 2 in, 2 out]
      }
      event "Test Name": Value Change {
        w370 = FALSE ("Visible")
        # "Tell the robot the test name to run"
        n221 = event-data() -> ("NewVal"=w374:u16)  [unwired: 1 in]
        n222 = property on="Test Name" class="Ring (strict)"() -> ("Strings []"=w375:string[])  [unwired: 2 in, 2 out]
        n223 = local write "Progress"(T4 {"Test Progress"=0, "Test Progress Text"=""} ("Progress")) -> ()
        n224 = Index Array(array=w375, index=w374) -> (element=w373:string)
        n225 = call <vilib>:"NT Write String.vi"("String"=w373, "Name"="TestMode/TestName") -> ()  [unwired: 9 in, 1 out]
        n226 = property on="Progress" class="Clust (strict)"("Visible"=TRUE) -> ()  [unwired: 2 in, 2 out]
        n227 = property on="Motor" class="Clust (strict)"("Visible"=w370) -> ()  [unwired: 2 in, 2 out]
        n228 = property on="Slider" class="Slide (strict)"("Visible"=w370) -> ()  [unwired: 2 in, 2 out]
        n229 = property on="On/Off" class="Bool (strict)"("Visible"=w370) -> ()  [unwired: 2 in, 2 out]
        n230 = property on="Rev/Fwd" class="Clust (strict)"("Visible"=w370) -> ()  [unwired: 2 in, 2 out]
        n231 = property on="Ring" class="Ring (strict)"("Visible"=w370) -> ()  [unwired: 2 in, 2 out]
      }
      event "Listbox": Double Click {
        n232 = event-data() -> ("PlatMods.Shift"=w378:bool, "Row"=w380:i32)  [unwired: 1 in]
        n233 = case shown="False" w378 {
          tunnel: w380 -> [w384 _]
          tunnel: 1 -> [w383 _]
          frame False {
            n234 = property on="Listbox" class="LstBox (strict)"() -> ("Item Symbols"=w382:i32[])  [unwired: 2 in, 2 out]
            n235 = Replace Array Subset(array=w382, new element=w383, index=w384) -> (w381:i32[])
            n236 = property on="Listbox" class="LstBox (strict)"("Item Symbols"=w381) -> ()  [unwired: 2 in, 2 out]
          }
          frame True {
            w385 = 0 ("Top Row")
            n237 = property on="Listbox" class="LstBox (strict)"() -> ("Number of Rows"=w387:u32)  [unwired: 2 in, 2 out]
            n238 = Initialize Array(0, w387) -> (w386:i32[])
            n239 = property on="Listbox" class="LstBox (strict)"("Top Row"=w385, "Value"=w385, "Item Symbols"=w386) -> ()  [unwired: 2 in, 2 out]
          }
        }
      }
      event "Listbox": Key Down {
        n240 = event-data() -> ("VKey"=w391:T19)  [unwired: 1 in]
        n241 = case shown="\"Left\", \"Right\"" w391 {
          selector: w391 -> [w396 _]
          tunnel: eventvkey."Left" ("VKey") -> [w394 _]
          frame "Left", "Right" {
            n242 = Equal?(x=w394, y=w396) -> (x = y?=w395:bool)
            n243 = Select(t=0, s=w395, f=1) -> (s? t:f=w397:i32)
            n244 = property on="Listbox" class="LstBox (strict)"() -> ("Item Symbols"=w400:i32[])  [unwired: 2 in, 2 out]
            n245 = Replace Array Subset(array=w400, new element=w397, index="Listbox") -> (w399:i32[])
            n246 = property on="Listbox" class="LstBox (strict)"("Item Symbols"=w399) -> ()  [unwired: 2 in, 2 out]
          }
          frame Default {
          }
        }
      }
      event "DB Camera Config": Value Change {
        n247 = event-data() -> ("NewVal"=w404:bool)  [unwired: 1 in]
        n248 = case shown="False" w404 {
          tunnel: w403 -> [w413 _]
          tunnel: [w406 w424] -> w402
          tunnel: w401 -> [w405 w424]
          frame False {
            w420 = "Camera"
            w423 = FALSE ("Visible")
            n249 = local read "Camera Settings"() -> (w412:T1)
            n250 = Index Array(array=w413) -> (element=w416:cluster{string[]})  [unwired: 1 in]
            n251 = Unbundle(w412) -> ("Frate Rate"=w411:i32, "Compression"=w410:i32, "Size"=w414:u16)
            n252 = Unbundle(w416) -> (w415:string[])
            n253 = Index Array(array=w415, index=w414) -> (element=w409:string)
            n254 = call-poly <vilib>:"Write Key.vi"("section"=w420, "value"=w409, "key"="Size", "refnum"=w405) -> ("refnum out"=w422:T18)  [unwired: 2 in, 5 out]
            n255 = call-poly <vilib>:"Write Key.vi"("section"=w420, "value"=w411, "key"="FrameRate", "refnum"=w422) -> ("refnum out"=w421:T18)  [unwired: 1 in, 6 out]
            n256 = property on="Camera Settings" class="Clust (strict)"("Visible"=w423) -> ()  [unwired: 2 in, 2 out]
            n257 = local write "DB Camera Config"(w423) -> ()
            n258 = call-poly <vilib>:"Write Key.vi"("section"=w420, "value"=w410, "key"="Compression", "refnum"=w421) -> ("refnum out"=w407:T18)  [unwired: 1 in, 6 out]
            n259 = call <vilib>:"Close Config Data.vi"("refnum"=w407) -> ("file path"=w408:path)  [unwired: 2 in, 8 out]
            n260 = call <vilib>:"Open Config Data.vi"("configuration file path"=w408) -> ("refnum"=w406:T18)  [unwired: 8 in, 2 out]
          }
          frame True {
            n261 = property on="Camera Settings" class="Clust (strict)"("Visible"=TRUE) -> ()  [unwired: 2 in, 2 out]
          }
        }
      }
      event "Camera Settings": Value Change {
        n262 = event-data() -> ("NewVal"=w437:T1)  [unwired: 1 in]
        n263 = Index Array(array=w433) -> (element=w432:cluster{string[]})  [unwired: 1 in]
        n264 = Unbundle(w437) -> ("Frate Rate"=w428:i32, "Compression"=w427:i32, "Size"=w430:u16)
        n265 = Unbundle(w432) -> (w431:string[])
        n266 = Index Array(array=w431, index=w430) -> (element=w429:string)
        n267 = Format Into String(format string="%s   %dfps   %d%%", w429, w428, w427) -> (resulting string=w434:string)  [unwired: 2 in, 1 out]
        n268 = Build Array(w434) -> (w435:string[])
        n269 = property on="DB Camera Config" class="Bool (strict)"("Strings [4]"=w435) -> ()  [unwired: 2 in, 2 out]
      }
      event "Motor.Enable": Value Change {
        n270 = event-data() -> ("NewVal"=w443:bool)  [unwired: 1 in]
        n271 = Unbundle("Motor") -> ("Value"=w442:dbl)  [unwired: 1 out]
        n272 = Select(t=w442, s=w443, f=0.0) -> (s? t:f=w440:dbl)
        n273 = call <vilib>:"NT Write Number.vi"("Numeric"=w440, "Name"=w439) -> ()  [unwired: 9 in, 1 out]
      }
      event "Slider": Value Change {
        n274 = event-data() -> ("NewVal"=w446:dbl)  [unwired: 1 in]
        n275 = call <vilib>:"NT Write Number.vi"("Numeric"=w446, "Name"=w447) -> ()  [unwired: 9 in, 1 out]
      }
      event "On/Off": Value Change {
        n276 = event-data() -> ("NewVal"=w451:bool)  [unwired: 1 in]
        n277 = Boolean To (0,1)(Boolean=w451) -> (0, 1=w450:i16)
        n278 = call <vilib>:"NT Write Number.vi"("Numeric"=w450, "Name"=w449) -> ()  [unwired: 9 in, 1 out]
      }
      event "Rev/Fwd": Value Change {
        n279 = event-data() -> ("NewVal.Forward"=w459:bool, "NewVal.Reverse"=w458:bool)  [unwired: 1 in]
        n280 = Boolean To (0,1)(Boolean=w459) -> (0, 1=w455:i16)
        n281 = Boolean To (0,1)(Boolean=w458) -> (0, 1=w457:i16)
        n282 = Negate(x=w457) -> (-x=w456:i16)
        n283 = Add(x=w455, y=w456) -> (x+y=w454:i16)
        n284 = call <vilib>:"NT Write Number.vi"("Numeric"=w454, "Name"=w453) -> ()  [unwired: 9 in, 1 out]
      }
      event "Ring": Value Change {
        n285 = event-data() -> ("NewVal"=w463:u16)  [unwired: 1 in]
        n286 = property on="Ring" class="Ring (strict)"() -> ("Strings []"=w464:string[])  [unwired: 2 in, 2 out]
        n287 = Index Array(array=w464, index=w463) -> (element=w462:string)
        n288 = call <vilib>:"NT Write String.vi"("String"=w462, "Name"=w461) -> ()  [unwired: 9 in, 1 out]
      }
    }
  }
  n289 = Index Array(array=w26) -> (element=w27:cluster{string[]})  [unwired: 1 in]
  n290 = Unbundle(w27) -> (w25:string[])
  n291 = Match First String(2:w25, 3:w24) -> (0:w23:i32)  [unwired: 1 out]
  n292 = Bundle("value"=w29, "value"=w28, "index"=w23) -> (w17:cluster{"value":i32, "value":i32, "index":i32})  [unwired: 1 out]
  n293 = disable-structure shown="Disabled" {
    frame Disabled {
      # "Terminals of controls and indicators\nthat are bound to the smart dashboard by name.\nYou can place them anywhere you like and\neven read data from them."
      n294 = call <vilib>:"Intialize Keyboard.vi"() -> ()  [unwired: 1 in, 11 out]
      n295 = call-poly <vilib>:"Acquire Input Data.vi"() -> ()  [unwired: 3 in, 17 out]
    }
    frame Enabled {
    }
  }
  n296 = property on="On/Off" class="Bool (strict)"("Visible"=w40) -> ()  [unwired: 2 in, 2 out]
  n297 = property on="Motor" class="Clust (strict)"("Visible"=w40) -> ()  [unwired: 2 in, 2 out]
  n298 = property on="Progress" class="Clust (strict)"("Visible"=w40) -> ()  [unwired: 2 in, 2 out]
  n299 = property on="Ring" class="Ring (strict)"("Visible"=w40) -> ()  [unwired: 2 in, 2 out]
  n300 = property on="Camera Settings" class="Clust (strict)"("Val(Sgnl)"=w17) -> ()  [unwired: 2 in, 2 out]
  n301 = property on="Rev/Fwd" class="Clust (strict)"("Visible"=w40) -> ()  [unwired: 2 in, 2 out]
  n302 = property on="Camera Settings" class="Clust (strict)"("Visible"=w40) -> ()  [unwired: 2 in, 2 out]
  n303 = local write "DB Camera Config"(w40) -> ()
